vi "Scale Front Panel Controls.vi"(8 "error in (no error)":errorcluster, 9 "Pane 2":refnum<vi>, 10 "Pane":refnum<vi>, 11 "Message Log in":refnum<class "Message Log.lvclass">) -> (0 "error out":errorcluster, 3 "Message Log out":refnum<class "Message Log.lvclass">)   [LabVIEW 2017, in "Message Log.lvclass"]
uses:
  Message Log.lvclass
  Message Log.lvclass/Message Log.ctl
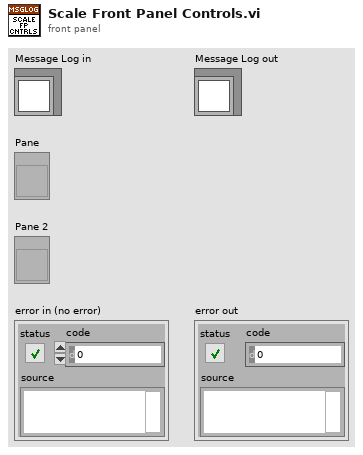
[diagram p1: front panel]
types:
  T1 = typedef "LVBoundsTypeDef.ctl" = cluster{"Width":u32, "Height":u32}
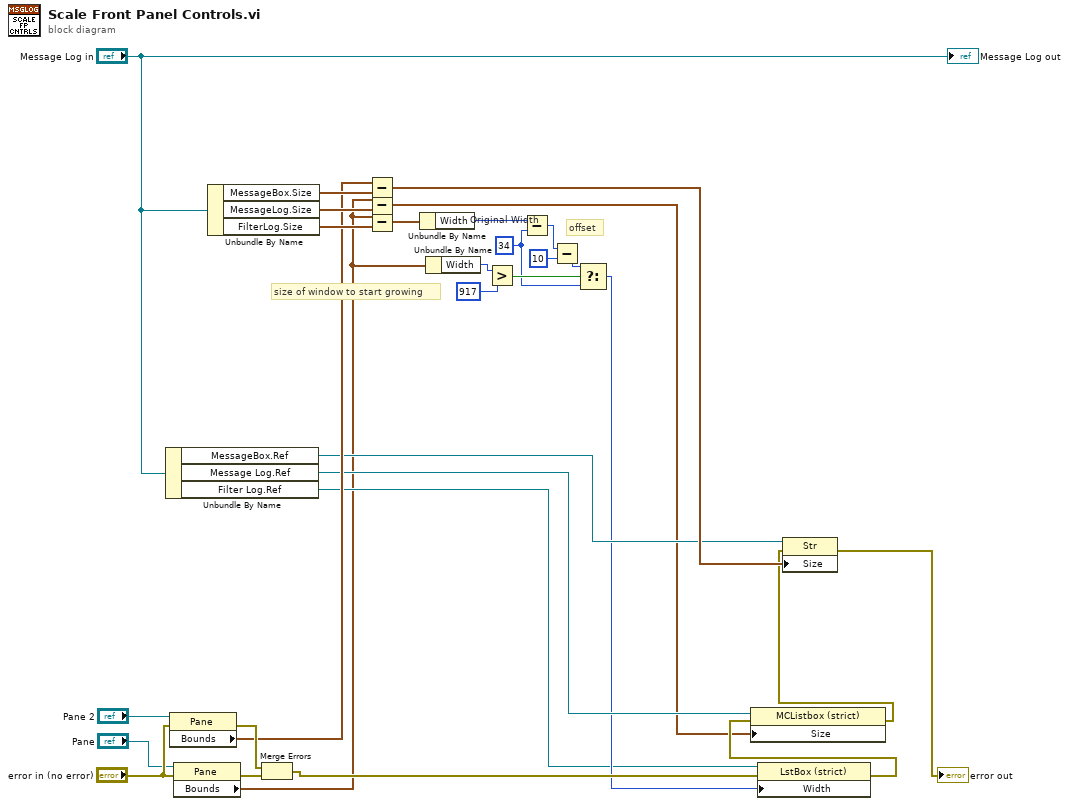
[diagram p0: block diagram]
diagram:
  w19 = u32 34  # Original Width
  # "offset"
  # "size of window to start growing"
  n1 = Unbundle By Name("Message Log in") -> ("MessageBox.Ref"=w7:refnum<vi>, "Message Log.Ref"=w6:refnum<vi>, "Filter Log.Ref"=w3:refnum<vi>)
  n2 = property class="Pane"(reference="Pane 2", error in="error in (no error)") -> (error out=w25:errorcluster, "Bounds"=w8:T1)  [unwired: 1 out]
  n3 = property class="Pane"(reference="Pane", error in="error in (no error)") -> (error out=w30:errorcluster, "Bounds"=w1:T1)  [unwired: 1 out]
  n4 = Unbundle By Name("Message Log in") -> ("MessageBox.Size"=w10:T1, "MessageLog.Size"=w9:T1, "FilterLog.Size"=w11:T1)
  n5 = Merge Errors(w25, w30) -> (w26:errorcluster)
  n6 = Subtract(x=w8, y=w10) -> (x-y=w28:T1)
  n7 = Subtract(x=w1, y=w9) -> (x-y=w5:T1)
  n8 = Subtract(x=w1, y=w11) -> (x-y=w23:T1)
  n9 = Unbundle By Name(w23) -> ("Width"=w18:u32)
  n10 = Unbundle By Name(w1) -> ("Width"=w22:u32)
  n11 = Greater?(x=w22, y=u32 917) -> (0:w20:bool)
  n12 = Subtract(x=w18, y=w19) -> (x-y=w17:u32)
  n13 = Subtract(x=w17, y=u32 10) -> (x-y=w16:u32)
  n14 = Select(t=w16, s=w20, f=w19) -> (s? t:f=w4:u32)
  n15 = property class="LstBox (strict)"(reference=w3, error in=w26, "Width"=w4) -> (error out=w24:errorcluster)  [unwired: 1 out]
  n16 = property class="MCListbox (strict)"(reference=w6, error in=w24, "Size"=w5) -> (error out=w12:errorcluster)  [unwired: 1 out]
  n17 = property class="Str"(reference=w7, error in=w12, "Size"=w28) -> (error out=→"error out":errorcluster)  [unwired: 1 out]
  "Message Log out" <- "Message Log in"
